vi "FM_Tx2012.vi"() -> ()   [LabVIEW 2014]
uses:
  <vilib>/Analysis/baseanly.llb/Quick Scale 1D.vi
  <vilib>/Analysis/3filter.llb/IIR Filter (DBL).vi
  <instrlib>/niUSRP/niUSRP Write Tx Data (CDB WDT).vi
  <vilib>/measure/NI_MAPro.lvlib
  <vilib>/Analysis/NI_AALBase.lvlib
panel:
  out "Message":waveform(dbl)(graph)
  out "error out":errorcluster
  in  "stop":bool
  in  "Peak deviation (Hz)":dbl=30000.0
  in  "#tones":i32=3
  in  "delta frequency":dbl=1000.0 format="%.2p"
  in  "start frequency":dbl=1000.0 format="%.2p"
  in  "message length (samples)":dbl=200000.0
  in  "active antenna":string="TX1"
  out "actual gain (dB)":dbl format="%#_6f"
  in  "gain (dB)":dbl format="%#_6f"
  out "actual carrier frequency":dbl=100000.0 format="%#_6p"
  in  "carrier frequency":dbl=915000000.0 format="%#_6p"
  out "actual IQ rate":dbl=100000.0 format="%#_6p"
  in  "IQ rate":dbl=1000000.0 format="%#_6p"
  in  "device names":refnum<k15>="192.168.10.2"
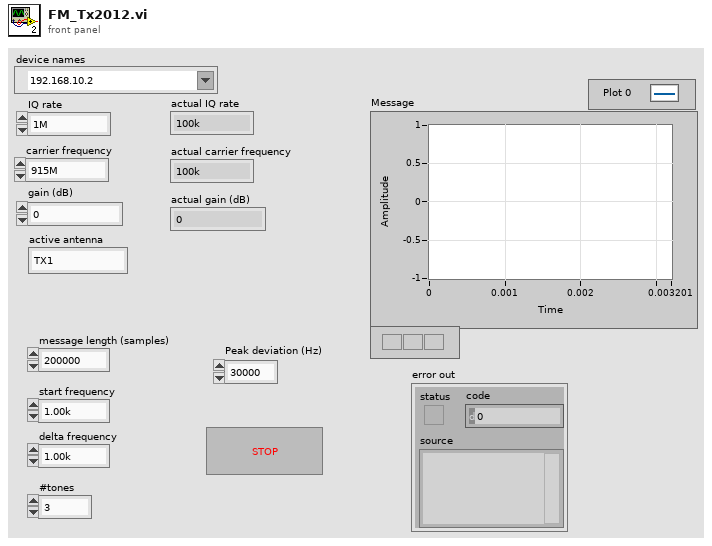
[diagram p1: front panel]
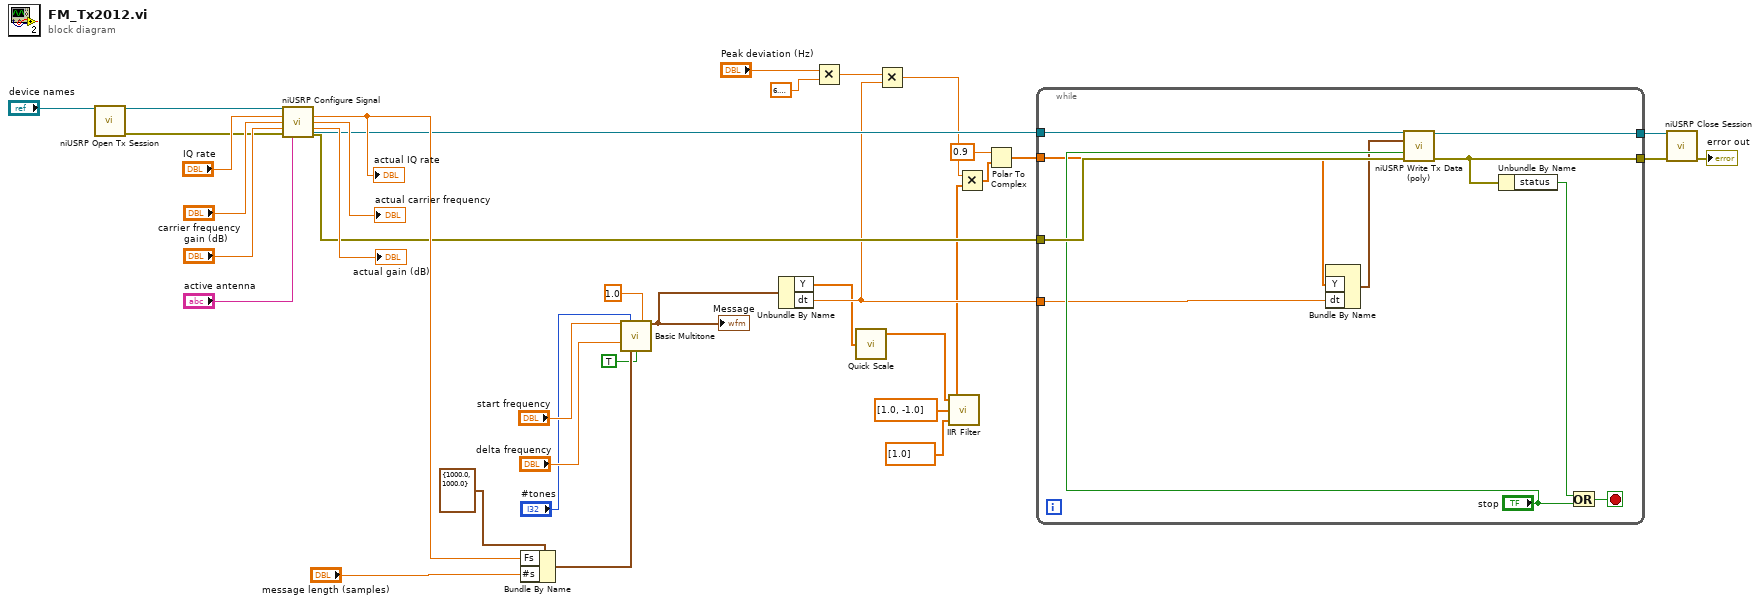
[diagram p0: block diagram]
diagram:
  n1 = call <instrlib>:"niUSRP Open Tx Session.vi"("device names"="device names") -> ("session handle out"=w36:refnum<k15>, "error out"=w30:errorcluster)  [unwired: 13 in]
  n2 = call <instrlib>:"niUSRP Configure Signal.vi"("session handle"=w36, "IQ rate"="IQ rate", "carrier frequency"="carrier frequency", "gain"="gain (dB)", "error in (no error)"=w30, "active antenna"="active antenna") -> ("session handle out"=w21:refnum<k15>, "coerced IQ rate"=w27:dbl, "coerced carrier frequency"=→"actual carrier frequency":dbl, "coerced gain"=→"actual gain (dB)":dbl, "error out"=w19:errorcluster)  [unwired: 5 in]
  "actual IQ rate" <- w27
  n3 = Bundle By Name(cluster=cluster{"Fs":dbl, "#s":dbl} {"Fs"=1000.0, "#s"=1000.0} ("sampling info"), "Fs"=w27, "#s"="message length (samples)") -> (w22:cluster{"Fs":dbl, "#s":dbl})
  n4 = call <vilib>:"Basic Multitone.vi"("start frequency"="start frequency", "#tones"="#tones", "amplitude"=1.0, "delta frequency"="delta frequency", "sampling info"=w22, "coerce frequencies?"=TRUE) -> ("signal out"=w15:waveform(dbl))  [unwired: 6 in, 3 out]
  "Message" <- w15
  n5 = Unbundle By Name(w15) -> ("Y"=w9:dbl[], "dt"=w11:dbl)
  n6 = Multiply(x="Peak deviation (Hz)", y=6.283185307179586) -> (x*y=w12:dbl)
  n7 = call-poly <vilib>:"Quick Scale.vi"("X"=w9) -> ("Y[i]=X[i]/Max|X|"=w6:dbl[])  [unwired: 2 out]
  n8 = Multiply(x=w12, y=w11) -> (x*y=w5:dbl)
  n9 = call-poly <vilib>:"IIR Filter.vi"("Forward Coefficients"=dbl[] [1.0], "Reverse Coefficients"=dbl[] [1.0, -1.0], "X"=w6) -> ("Filtered X"=w4:dbl[])  [unwired: 1 in, 1 out]
  n10 = Multiply(x=w5, y=w4) -> (x*y=w2:dbl[])
  n11 = Polar To Complex(1:w2, 2:0.9 ("r")) -> (0:w1:cdb[])
  n12 = while {
    tunnel: w21 -> [w47]
    tunnel: [w46] -> w20
    tunnel: w19 -> [w45]
    tunnel: [w41] -> w18
    tunnel: w11 -> [w40]
    tunnel: w1 -> [w38]
    stop <- w43 stop-if-true
    n13 = Bundle By Name("Y"=w38, "dt"=w40) -> (w39:waveform(cdb))  [unwired: 1 in]
    n14 = call-poly <instrlib>:"niUSRP Write Tx Data (poly).vi"("session handle"=w47, "data"=w39, "end of data?"="stop", "error in (no error)"=w45) -> ("session handle out"=w46:refnum<k15>, "error out"=w41:errorcluster)  [unwired: 10 in]
    n15 = Unbundle By Name(w41) -> ("status"=w44:bool)
    n16 = Or(x=w44, y="stop") -> (x .or. y?=w43:bool)
  }
  n17 = call <instrlib>:"niUSRP Close Session.vi"("session handle"=w20, "error in (no error)"=w18) -> ("error out"=→"error out":errorcluster)  [unwired: 13 in]
